vi "Fill.vi"(3 "Error":string, 4 "Value":u8, 5 "Image":T1={"Image ID"=0, "Channel ID"=-1}) -> (0 "Error":string, 2 "Image":T1={"Image ID"=0, "Channel ID"=-1})   [LabVIEW 2011, in "labvvis.lvlib"]
doc: "Sets all pixels in Image to Value. If Image is an RGBA image, all the channels of the image are set to Value. Thus this VI will only fill a RGBA image with grey pixels."
uses:
  <userlib>/labvvis/labvvis.lvlib
  <userlib>/labvvis/VVIS Image.ctl
  labvvis.framework
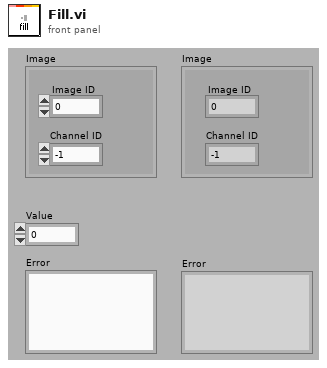
[diagram p1: front panel]
types:
  T1 = typedef "labvvis.lvlib/VVIS Image.ctl" = cluster{"Image ID":i16, "Channel ID":i16}
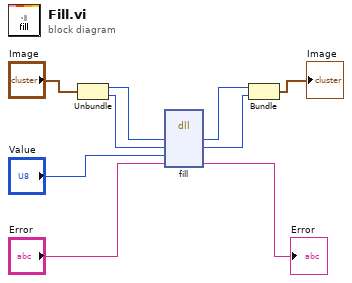
[diagram p0: block diagram]
diagram:
  n1 = Unbundle("Image") -> ("Image ID"=w8:i16, "Channel ID"=w3:i16)
  n2 = dll-call lib="labvvis.framework" fn="fill"("out"=w8, "out_ch"=w3, "value"="Value", "error"="Error") -> ("out"=w7:i16, "out_ch"=w4:i16, "error"=→"Error":string)  [unwired: 5 in, 2 out]
  n3 = Bundle("out"=w7, "out_ch"=w4) -> (→"Image":cluster{"out":i16, "out_ch":i16})  [unwired: 1 in]
